vi "Test Multiple IDs Client.vi"() -> ()   [LabVIEW 2020, in "Test.lvlib"]
uses:
  Test.lvlib
  TCP Comms/State.ctl
  Slider ID.ctl
  0ccc8330-39ba-48a1-8223-cf5070bef32b.vi
  56c8a86d-a319-4de7-adfb-b6a856ff4293.vi
  259ed48f-7e9e-4079-aa69-b33d26c51f3a.vi
  <vilib>/Utility/error.llb/Clear Errors.vi
  TCP Comms/Get Connected.vi
  <vilib>/Utility/error.llb/Error Cluster From Error Code.vi
  TCP Comms/Connection Ref.vi
  TCP Comms/Close TCP.vi
  TCP Comms/TinyTCP.lvlib
panel:
  in  "Close":bool
  in  "Open":bool
  out "Client State":T1
  out "Slider D (Server)":i8(slide) scale=0.0..10.0
  out "Slider C (Server)":u16(slide) scale=0.0..10.0
  in  "Slider B (Client)":dbl(slide) scale=0.0..10.0
  in  "Slider A (Client)":i32(slide) scale=0.0..10.0
  # "Close the window to stop the client"
  # "Run this VI and then click Open Client to open the connection to the server. Connections can be open in any order and once the connection is established, the values will start being sent to and read from the connected server.\n\nClose Client closes the connection but leaves the app running and the client can be opened again."
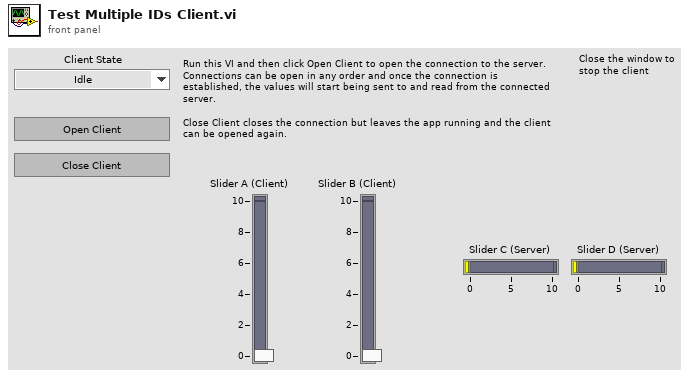
[diagram p1: front panel]
types:
  T1 = typedef "TinyTCP.lvlib/State.ctl" = enum16{"Idle", "Starting", "Connecting", "Connected", "Disconnecting", "Stopped"}
  T2 = typedef "TinyTCP.lvlib/Instance.ctl" = refnum<data-value>
  T3 = typedef "Test.lvlib/Slider ID.ctl" = enum16{"Slider A", "Slider B", "Slider C", "Slider D"}
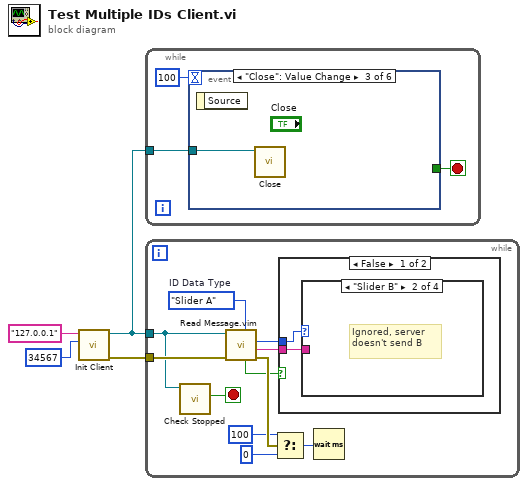
[diagram p0: block diagram]
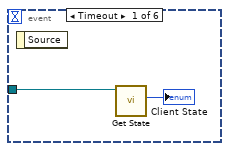
[diagram p2: hidden frame]
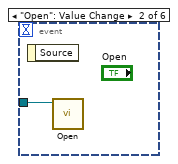
[diagram p3: hidden frame]
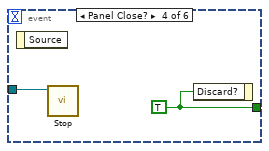
[diagram p4: hidden frame]
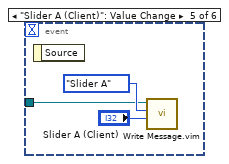
[diagram p5: hidden frame]
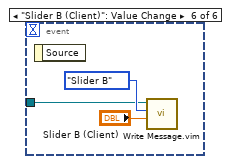
[diagram p6: hidden frame]
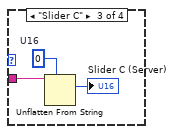
[diagram p8: hidden frame]
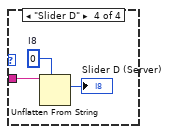
[diagram p9: hidden frame]
diagram:
  n1 = call "Init Client.vi"("Port"=u16 34567, "Host"="127.0.0.1") -> ("error out"=w4:errorcluster, "TinyTCP Client"=w1:T2)  [unwired: 8 in]
  n2 = while {
    tunnel: w1 -> [w7]
    stop <- w6 stop-if-true
    n3 = event shown="[2] \"Close\": Value Change" {
      selector: _ -> [_ _ _ _ _ _]
      dyn-events: _ -> [_ _ _ _ _ _]
      timeout: 100 -> [_ _ _ _ _ _]
      tunnel: w7 -> [w9 w10 w11 w13 w14 w17]
      tunnel: [_ _ _ w12 _ _] -> w6
      event Timeout {
        n4 = event-data() -> ()  [unwired: 1 in, 1 out]
        n5 = call "Get State.vi"("TCP Comm In"=w9) -> ("State"=→"Client State":T1)  [unwired: 9 in, 1 out]
      }
      event "Open": Value Change {
        n6 = event-data() -> ()  [unwired: 1 in, 1 out]
        n7 = call "Open.vi"("TCP Comm"=w10) -> ()  [unwired: 10 in, 1 out]
      }
      event "Close": Value Change {
        n8 = event-data() -> ()  [unwired: 1 in, 1 out]
        n9 = call "Close.vi"("TCP Comm"=w11) -> ()  [unwired: 10 in, 1 out]
      }
      event Panel Close? {
        w12 = TRUE
        n10 = event-data() -> ()  [unwired: 1 in, 1 out]
        n11 = call "Stop.vi"("TCP Comm"=w13) -> ()  [unwired: 10 in, 1 out]
        n12 = event-data("Discard?"=w12) -> ()  [unwired: 1 in, 1 out]
      }
      event "Slider A (Client)": Value Change {
        n13 = event-data() -> ()  [unwired: 1 in, 1 out]
        n14 = call "Write Message.vim"("Data"="Slider A (Client)", "Message ID (None)"=Slider_ID."Slider A" ("Slider ID"), "TCP Comm In"=w14) -> ()  [unwired: 6 in, 3 out]
      }
      event "Slider B (Client)": Value Change {
        n15 = event-data() -> ()  [unwired: 1 in, 1 out]
        n16 = call "Write Message.vim"("Data"="Slider B (Client)", "Message ID (None)"=Slider_ID."Slider B" ("Slider ID"), "TCP Comm In"=w17) -> ()  [unwired: 6 in, 3 out]
      }
    }
  }
  n17 = while {
    tunnel: w1 -> [w20]
    tunnel: w4 -> [w29]
    stop <- w21 stop-if-true
    w28 = Slider_ID."Slider A"  # ID Data Type
    n18 = call "Check Stopped.vi"("TCP Comm In"=w20) -> ("Stopped?"=w21:bool)  [unwired: 9 in, 1 out]
    n19 = call "Read Message.vim"("Message ID Data Type (String)"=w28, "error in (no error)"=w29, "TCP Comm In"=w20) -> ("error out"=w30:errorcluster, "Data"=w25:string, "Message ID"=w26:T3, "Timeout?"=w27:bool)  [unwired: 3 in, 2 out]
    n20 = Select(t=u32 100, s=w30, f=u32 0 ("milliseconds to wait")) -> (s? t:f=w23:u32)
    n21 = case shown="False" w27 {
      tunnel: w26 -> [w32 _]
      tunnel: w25 -> [w31 _]
      frame False {
        n22 = case shown="\"Slider B\"" w32 {
          tunnel: w31 -> [_ _ w35 w37]
          frame "Slider A" {
            # "Ignored, server doesn't send A"
          }
          frame "Slider B" {
            # "Ignored, server doesn't send B"
          }
          frame "Slider C" {
            w33 = u16 0  # U16
            n23 = Unflatten From String(type=w33, binary string=w35) -> (value=→"Slider C (Server)":u16)  [unwired: 3 in, 2 out]
          }
          frame "Slider D" {
            w38 = i8 0  # I8
            n24 = Unflatten From String(type=w38, binary string=w37) -> (value=→"Slider D (Server)":i8)  [unwired: 3 in, 2 out]
          }
        }
      }
      frame True {
      }
    }
    n25 = Wait (ms)(milliseconds to wait=w23) -> ()  [unwired: 1 out]
  }
